vi "19052 Get_Result_ALL_JUDGMENT.vi"(8 "error in (no error)":errorcluster, 11 "VISA resource in":refnum<visa-resource-name>) -> (0 "error out":errorcluster, 1 "JUDGMENT":string, 3 "VISA resource out":refnum<visa-resource-name>)   [LabVIEW 2015]
doc: "This VI obtains the mode of a selected step."
panel:
  out "output command":string
  # "Get Result ALL JUDGMENT"
  # "This is valid for both:\n19572 & 19052"
  # "Results after test"
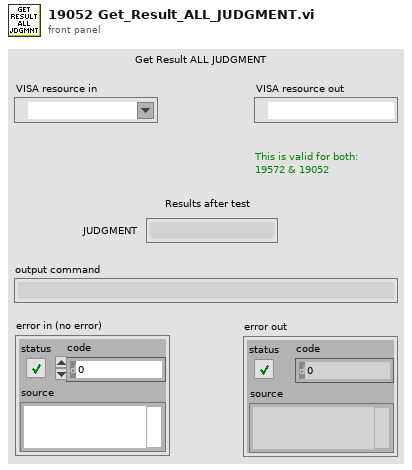
[diagram p1: front panel]
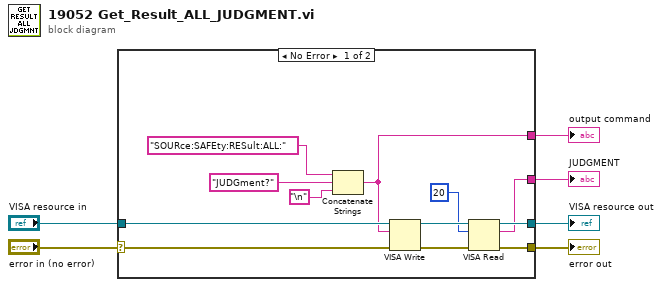
[diagram p0: block diagram]
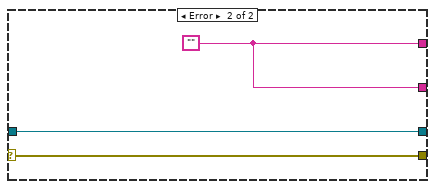
[diagram p2: hidden frame]
diagram:
  n1 = case shown="No Error" "error in (no error)" {
    selector: "error in (no error)" -> [w8 w20]
    tunnel: [w18 w20] -> w6
    tunnel: "VISA resource in" -> [w17 w21]
    tunnel: [w14 w19] -> w4
    tunnel: [w10 w21] -> w3
    tunnel: [w9 w19] -> w2
    frame No Error {
      n2 = Concatenate Strings("SOURce:SAFEty:RESult:ALL:", "JUDGment?", "\n") -> (w14:string)
      n3 = VISA Write(VISA resource name=w17, write buffer=w14, error in (no error)=w8) -> (VISA resource name out=w12:refnum<visa-resource-name>, error out=w13:errorcluster)  [unwired: 1 out]
      n4 = VISA Read(VISA resource name=w12, byte count=u32 20, error in (no error)=w13) -> (VISA resource name out=w10:refnum<visa-resource-name>, read buffer=w9:string, error out=w18:errorcluster)  [unwired: 1 out]
    }
    frame Error {
      w19 = ""
    }
  }
  "error out" <- w6
  "VISA resource out" <- w3
  "output command" <- w4
  "JUDGMENT" <- w2
